vi "DRAW_Mouse_track.vi"(0 "Image ref. in":T1, 1 "Trace color":u32, 2 "Trace color 2":u32, 5 "Track array in":cluster{"X":dbl, "Y":dbl}[](array[cluster]), 7 "Speed array in":dbl[](array[numeric]), 9 "Colors array input":u32[](array[colorbox]), 11 "Error In (no error)":errorcluster, 12 "Rainbow colors":bool, 13 "Bright mouse lineout":bool, 14 "Rainbow track is speed":bool) -> (4 "Image ref. out":T1, 15 "Error Out":errorcluster)   [LabVIEW 2018, in "Tracker.lvlib"]
uses:
  Tracker.lvlib
  <vilib>/vision/Image Controls.llb/IMAQ Image.ctl
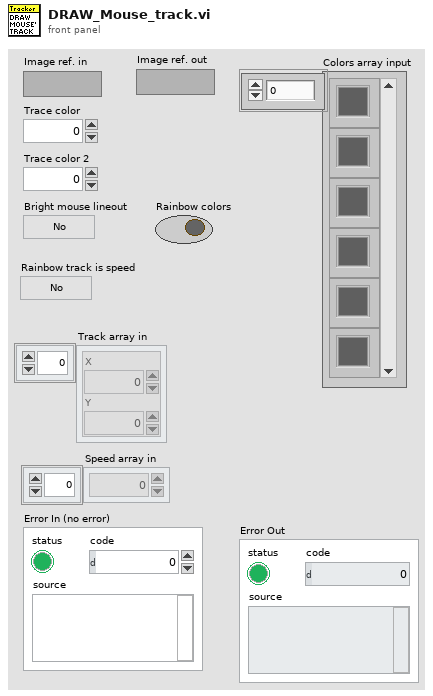
[diagram p1: front panel]
types:
  T1 = typedef "IMAQ Image.ctl" = refnum<image>
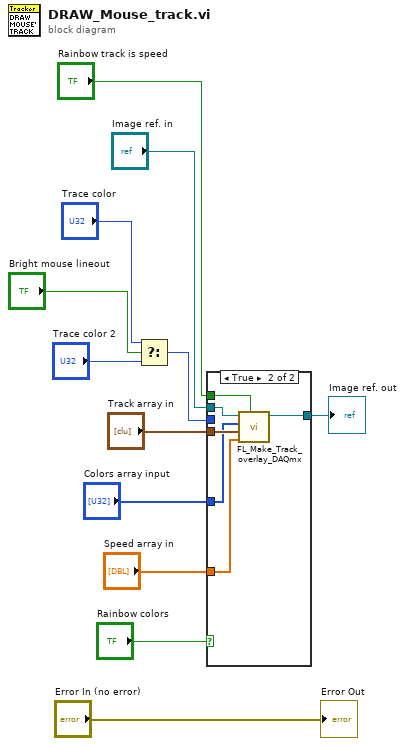
[diagram p0: block diagram]
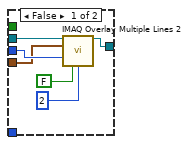
[diagram p2: hidden frame]
diagram:
  n1 = Select(t="Trace color", s="Bright mouse lineout", f="Trace color 2") -> (s? t:f=w8:u32)
  n2 = case shown="True" "Rainbow colors" {
    tunnel: w8 -> [w16 _]
    tunnel: "Track array in" -> [w15 w20]
    tunnel: "Image ref. in" -> [w18 w24]
    tunnel: [w17 w23] -> w12
    tunnel: "Speed array in" -> [_ w22]
    tunnel: "Rainbow track is speed" -> [_ w21]
    tunnel: "Colors array input" -> [_ w19]
    frame False {
      n3 = call "IMAQ Overlay Multiple Lines 2"("Image"=w18, "Line End Points"=w15, "Color"=w16, "Maintain Width?"=FALSE, "Width"=u32 2) -> ("Image Out"=w17:T1)  [unwired: 9 in, 1 out]
    }
    frame True {
      n4 = call "FL_Make_Track_overlay_DAQmx.vi"("Rainbow track is speed (F)"=w21, "Speed array"=w22, "Full track array"=w20, "Colors array input"=w19, "Image In"=w24) -> ("Image Out"=w23:T1)  [unwired: 3 in]
    }
  }
  "Image ref. out" <- w12
  "Error Out" <- "Error In (no error)"
